vi "Close Connection.vi"(8 "error in (no error)":errorcluster, 11 "RemoteControl.STM in":refnum<class "RemoteControl.STM.lvclass">) -> (0 "error out":errorcluster, 3 "RemoteControl.STM out":refnum<class "RemoteControl.STM.lvclass">)   [LabVIEW 2019, in "RemoteControl.STM.lvclass"]
uses:
  RemoteControl.STM.lvclass
  <vilib>/NI/STM/TCP/TCP Connection Info.ctl
  <vilib>/NI/STM/SubVIs/MetaDataElement.ctl
  RemoteControl.STM.lvclass/RemoteControl.STM.ctl
  <vilib>/NI/STM/TCP/Get Connection Reference (TCP).vi
  <userlib>/LevyLab/RemoteControl/RemoteControl.lvclass
  <vilib>/NI/STM/NI STM.lvlib
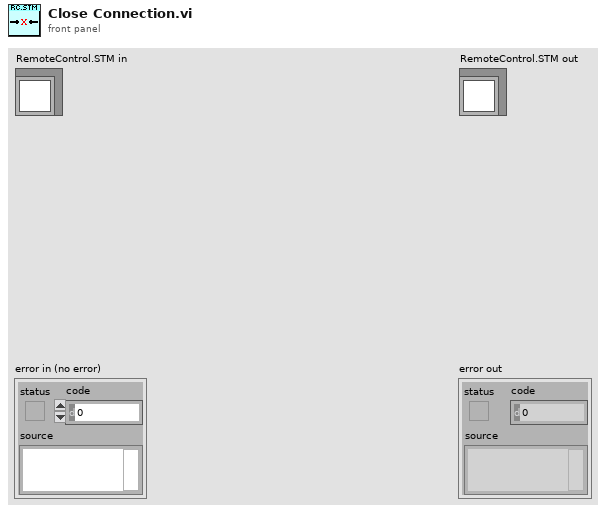
[diagram p1: front panel]
types:
  T1 = typedef "NI STM.lvlib/TCP Connection Info.ctl" = cluster{"connection ID":refnum<k5>, "meta data":T2[]}
  T2 = typedef "NI STM.lvlib/MetaDataElement.ctl" = string
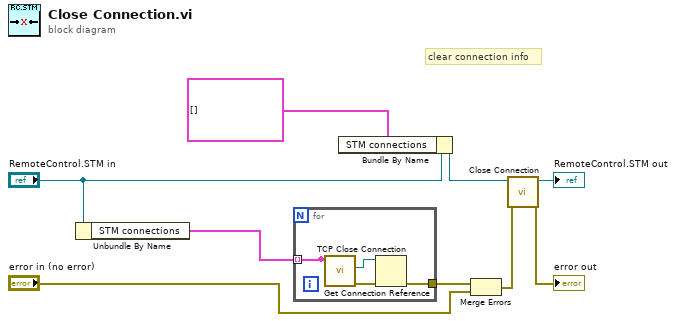
[diagram p0: block diagram]
diagram:
  # "clear connection info"
  n1 = Unbundle By Name("RemoteControl.STM in") -> ("STM connections"=w7:T1[])
  n2 = for {
    tunnel: [w10] -> _ mode=indexing
    tunnel: w7 -> [w10] mode=indexing
    tunnel: [w11] -> w3
    n3 = call-poly <vilib>:"Get Connection Reference.vi"("connection info in"=w10) -> ("error out"=w12:errorcluster, "connection ID out"=w13:refnum<k5>)  [unwired: 8 in, 1 out]
    n4 = TCP Close Connection(connection ID=w13, error in (no error)=w12) -> (error out=w11:errorcluster)  [unwired: 1 in, 1 out]
  }
  n5 = Bundle By Name(cluster="RemoteControl.STM in", "STM connections"=T1[] [] ("STM connection info")) -> (w6:refnum<class "RemoteControl.STM.lvclass">)
  n6 = Merge Errors(w3, "error in (no error)") -> (w2:errorcluster)
  n7 = call-parent "Close Connection.vi"("error in (no error)"=w2, "RemoteControl in"=w6) -> ("error out"=→"error out":errorcluster, "RemoteControl out"=→"RemoteControl.STM out":refnum<class "RemoteControl.STM.lvclass">)  [unwired: 8 in]
